vi "Read rx regs.vi"(11 "niUSRP Rx Core v1 FPGA in":refnum<class "niUSRP Rx Core v1 FPGA.lvclass">=refnum) -> (2 "rx regs":T1={"enable"="", "reset"="", "channel no."=0, "sample clock domain"="Data Clock", "i in resource"="RF 0/Rx/I", "q in resource"="", "Number of Chs"=0, "debug"="", "Loopback FIFO"="Loopback FIFO"}, 3 "niUSRP Rx Core v1 FPGA out":refnum<class "niUSRP Rx Core v1 FPGA.lvclass">)   [LabVIEW 2023]
uses:
  <instrlib>/niUSRP/Reference FPGA/Rx Core/niUSRP Rx Core v1 FPGA.lvclass
  <instrlib>/niUSRP/Reference FPGA/Rx Core/Regs.ctl
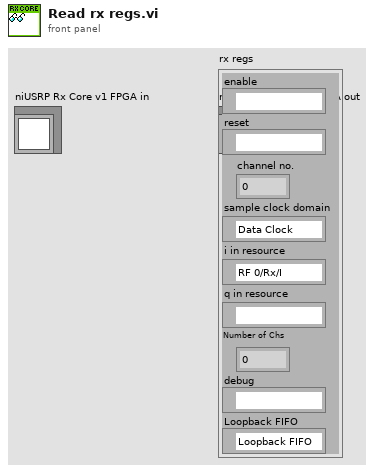
[diagram p1: front panel]
types:
  T1 = typedef "niUSRP Rx Core v1 FPGA.lvclass/Regs.ctl" = cluster{"enable":refnum<k21>, "reset":refnum<k21>, "channel no.":u8, "sample clock domain":refnum<k21>, "i in resource":refnum<k21>, "q in resource":refnum<k21>, "Number of Chs":u8, "debug":refnum<k21>, "Loopback FIFO":refnum<k21>}
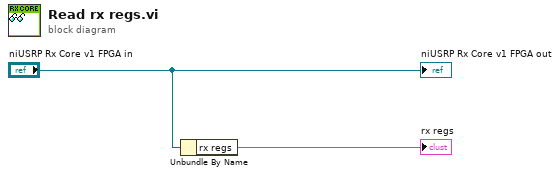
[diagram p0: block diagram]
diagram:
  n1 = Unbundle By Name("niUSRP Rx Core v1 FPGA in") -> ("rx regs"=→"rx regs")
  "niUSRP Rx Core v1 FPGA out" <- "niUSRP Rx Core v1 FPGA in"
